vi "AO Python Gen Fake Image.vi"(7 "Size (pixels)":i32=256) -> (8 "Fake Image":dbl[][][](array[numeric]))   [LabVIEW 2016]
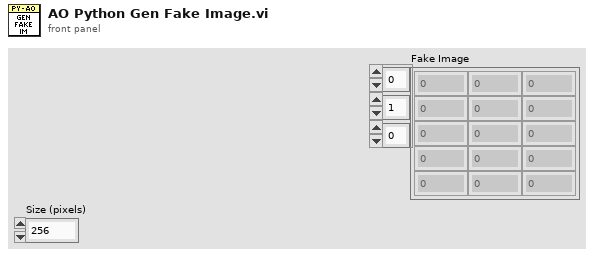
[diagram p1: front panel]
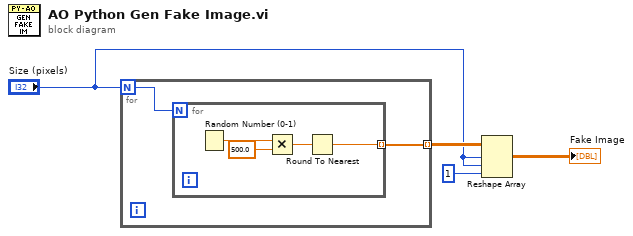
[diagram p0: block diagram]
diagram:
  n1 = for {
    N: "Size (pixels)" -> [w6]
    tunnel: [w5] -> w4 mode=indexing
    n2 = for {
      N: w6 -> [_]
      tunnel: [w7] -> w5 mode=indexing
      n3 = Random Number (0-1)() -> (number: 0 to 1=w10:dbl)
      n4 = Multiply(x=w10, y=500.0) -> (x*y=w8:dbl)
      n5 = Round To Nearest(number=w8) -> (nearest integer value=w7:dbl)
    }
  }
  n6 = Reshape Array(w4, "Size (pixels)", "Size (pixels)", 1 ("dimension size")) -> (→"Fake Image":dbl[][][])
